vi "rethinkdb_json_tokenize_next.vi"(9 "offset (0)":i32, 11 "json":string) -> (1 "offset past token":i32, 2 "arg":string, 3 "token":T1)   [LabVIEW 2017]
uses:
  rethinkdb_json_token.ctl
  <vilib>/regexp/Match Regular Expression.xnode
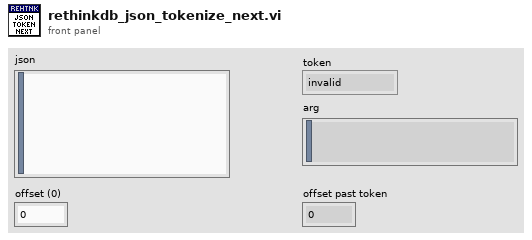
[diagram p1: front panel]
types:
  T1 = typedef "rethinkdb_json_token.ctl" = enum8{"invalid", "null", "boolean", "decimal", "float", "string", "key", "comma", "object_start", "object_end", "array_start", "array_end", "end"}
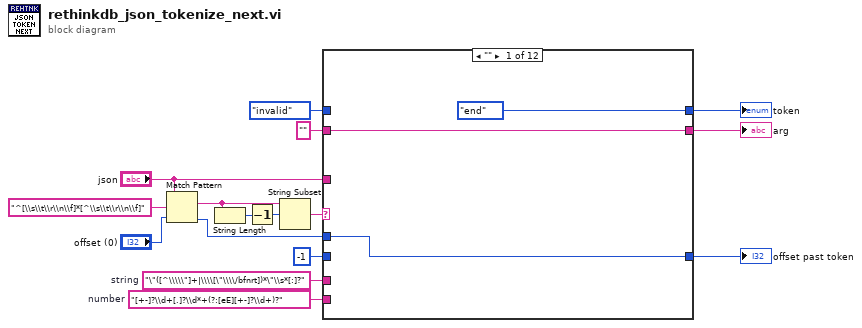
[diagram p0: block diagram]
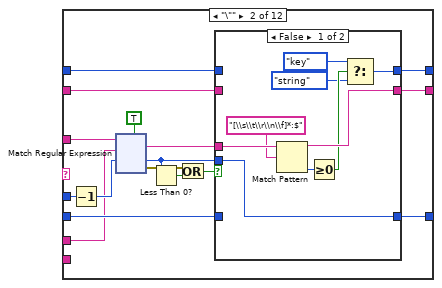
[diagram p2: hidden frame]
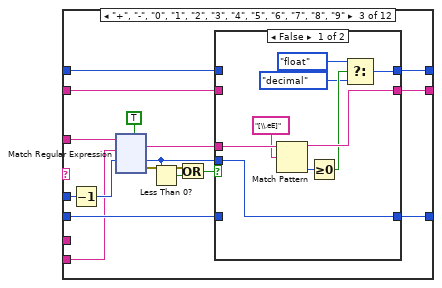
[diagram p4: hidden frame]
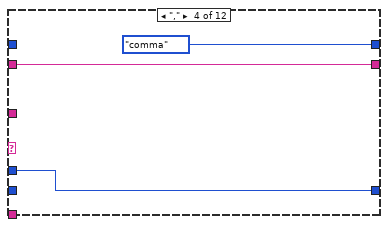
[diagram p6: hidden frame]
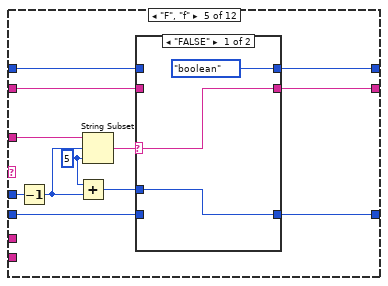
[diagram p7: hidden frame]
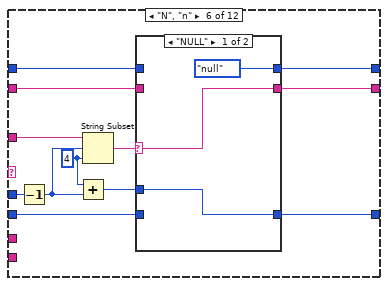
[diagram p9: hidden frame]
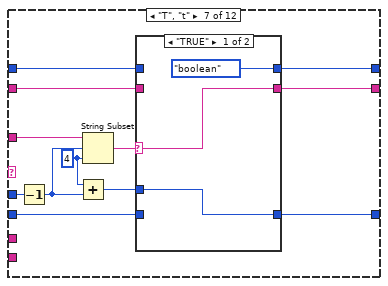
[diagram p11: hidden frame]
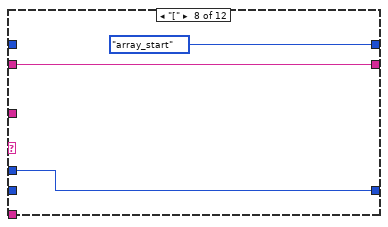
[diagram p13: hidden frame]
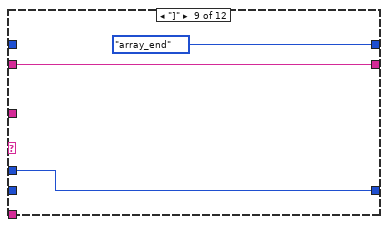
[diagram p14: hidden frame]
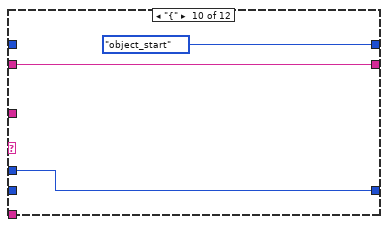
[diagram p15: hidden frame]
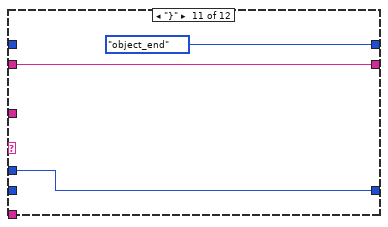
[diagram p16: hidden frame]
diagram:
  w1 = "[+-]?\\d+[.]?\\d*+(?:[eE][+-]?\\d+)?"  # number
  w2 = "\"([^\\\\\"]+|\\\\[\"\\\\/bfnrt])*\"\\s*[:]?"  # string
  n1 = Match Pattern(string="json", regular expression="^[\\s\\t\\r\\n\\f]*[^\\s\\t\\r\\n\\f]", offset (0)="offset (0)") -> (match substring=w13:string, offset past match=w8:i32)  [unwired: 2 out]
  n2 = String Length(string=w13) -> (length=w14:i32)
  n3 = Decrement(x=w14) -> (x-1=w12:i32)
  n4 = String Subset(string=w13, offset (0)=w12) -> (substring=w11:string)  [unwired: 1 in]
  n5 = case shown="\"\"" w11 {
    tunnel: [rethinkdb_json_token."end" ("token") w24 w166 rethinkdb_json_token."comma" ("token") w308 w326 w344 rethinkdb_json_token."array_start" ("token") rethinkdb_json_token."array_end" ("token") rethinkdb_json_token."object_start" ("token") rethinkdb_json_token."object_end" ("token") w375] -> w10
    tunnel: rethinkdb_json_token."invalid" ("token") -> [_ w23 w165 _ w307 w325 w343 _ _ _ _ w375]
    tunnel: w8 -> [w17 w33 w175 w304 w317 w335 w353 w361 w364 w367 w370 _]
    tunnel: [w17 w28 w170 w304 w312 w330 w348 w361 w364 w367 w370 w374] -> w7
    tunnel: -1 ("offset past match") -> [_ w27 w169 _ w311 w329 w347 _ _ _ _ w374]
    tunnel: [w19 w26 w168 w306 w310 w328 w346 w363 w366 w369 w372 w373] -> w5
    tunnel: "" -> [w19 w25 w167 w306 w309 w327 w345 w363 w366 w369 w372 w373]
    tunnel: "json" -> [_ w35 w177 _ w318 w336 w354 _ _ _ _ _]
    tunnel: w2 -> [_ w20 _ _ _ _ _ _ _ _ _ _]
    tunnel: w1 -> [_ _ w162 _ _ _ _ _ _ _ _ _]
    frame "" {
    }
    frame "\"" {
      n6 = Decrement(x=w33) -> (x-1=w32:i32)
      n7 = xnode "Match Regular Expression"("input string"=w35, "regular expression"=w20, "offset (0)"=w32, "multiline? (F)"=TRUE) -> ("whole match"=w21:string, "offset past match"=w22:i32, "error out"=w31:errorcluster)  [unwired: 2 in, 2 out]
      n8 = Less Than 0?(x=w22) -> (x < 0?=w30:bool)
      n9 = Or(x=w31, y=w30) -> (x .or. y?=w29:bool)
      n10 = case shown="False" w29 {
        tunnel: [w36 w47] -> w28
        tunnel: w27 -> [_ w47]
        tunnel: [w42 w46] -> w26
        tunnel: w25 -> [_ w46]
        tunnel: [w37 w45] -> w24
        tunnel: w23 -> [_ w45]
        tunnel: w22 -> [w36 _]
        tunnel: w21 -> [w44 _]
        frame False {
          n11 = Match Pattern(string=w44, regular expression="[\\s\\t\\r\\n\\f]*:$") -> (before substring=w42:string, offset past match=w41:i32)  [unwired: 1 in, 2 out]
          n12 = Greater Or Equal To 0?(x=w41) -> (x >= 0?=w40:bool)
          n13 = Select(t=rethinkdb_json_token."key" ("token"), s=w40, f=rethinkdb_json_token."string" ("token")) -> (s? t:f=w37:T1)
        }
        frame True {
        }
      }
    }
    frame "+", "-", "0", "1", "2", "3", "4", "5", "6", "7", "8", "9" {
      n14 = Decrement(x=w175) -> (x-1=w174:i32)
      n15 = xnode "Match Regular Expression"("input string"=w177, "regular expression"=w162, "offset (0)"=w174, "multiline? (F)"=TRUE) -> ("whole match"=w163:string, "offset past match"=w164:i32, "error out"=w173:errorcluster)  [unwired: 2 in, 2 out]
      n16 = Less Than 0?(x=w164) -> (x < 0?=w172:bool)
      n17 = Or(x=w173, y=w172) -> (x .or. y?=w171:bool)
      n18 = case shown="False" w171 {
        tunnel: [w178 w189] -> w170
        tunnel: w169 -> [_ w189]
        tunnel: [w184 w188] -> w168
        tunnel: w167 -> [_ w188]
        tunnel: [w179 w187] -> w166
        tunnel: w165 -> [_ w187]
        tunnel: w164 -> [w178 _]
        tunnel: w163 -> [w186 _]
        frame False {
          n19 = Match Pattern(string=w186, regular expression="[\\.eE]") -> (before substring=w184:string, offset past match=w183:i32)  [unwired: 1 in, 2 out]
          n20 = Greater Or Equal To 0?(x=w183) -> (x >= 0?=w182:bool)
          n21 = Select(t=rethinkdb_json_token."float" ("token"), s=w182, f=rethinkdb_json_token."decimal" ("token")) -> (s? t:f=w179:T1)
        }
        frame True {
        }
      }
    }
    frame "," {
    }
    frame "F", "f" {
      w315 = 5 ("length (rest)")
      n22 = Decrement(x=w317) -> (x-1=w316:i32)
      n23 = Add(x=w315, y=w316) -> (x+y=w314:i32)
      n24 = String Subset(string=w318, offset (0)=w316, length (rest)=w315) -> (substring=w313:string)
      n25 = case shown="\"FALSE\"" w313 {
        selector: w313 -> [w320 _]
        tunnel: w314 -> [w319 _]
        tunnel: [w319 w324] -> w312
        tunnel: w311 -> [_ w324]
        tunnel: [w320 w323] -> w310
        tunnel: w309 -> [_ w323]
        tunnel: [rethinkdb_json_token."boolean" ("token") w322] -> w308
        tunnel: w307 -> [_ w322]
        frame "FALSE" {
        }
        frame Default {
        }
      }
    }
    frame "N", "n" {
      w333 = 4 ("length (rest)")
      n26 = Decrement(x=w335) -> (x-1=w334:i32)
      n27 = Add(x=w333, y=w334) -> (x+y=w332:i32)
      n28 = String Subset(string=w336, offset (0)=w334, length (rest)=w333) -> (substring=w331:string)
      n29 = case shown="\"NULL\"" w331 {
        selector: w331 -> [w338 _]
        tunnel: w332 -> [w337 _]
        tunnel: [w337 w342] -> w330
        tunnel: w329 -> [_ w342]
        tunnel: [w338 w341] -> w328
        tunnel: w327 -> [_ w341]
        tunnel: [rethinkdb_json_token."null" ("token") w340] -> w326
        tunnel: w325 -> [_ w340]
        frame "NULL" {
        }
        frame Default {
        }
      }
    }
    frame "T", "t" {
      w351 = 4 ("length (rest)")
      n30 = Decrement(x=w353) -> (x-1=w352:i32)
      n31 = Add(x=w351, y=w352) -> (x+y=w350:i32)
      n32 = String Subset(string=w354, offset (0)=w352, length (rest)=w351) -> (substring=w349:string)
      n33 = case shown="\"TRUE\"" w349 {
        selector: w349 -> [w356 _]
        tunnel: w350 -> [w355 _]
        tunnel: [w355 w360] -> w348
        tunnel: w347 -> [_ w360]
        tunnel: [w356 w359] -> w346
        tunnel: w345 -> [_ w359]
        tunnel: [rethinkdb_json_token."boolean" ("token") w358] -> w344
        tunnel: w343 -> [_ w358]
        frame "TRUE" {
        }
        frame Default {
        }
      }
    }
    frame "[" {
    }
    frame "]" {
    }
    frame "{" {
    }
    frame "}" {
    }
    frame Default {
    }
  }
  "token" <- w10
  "arg" <- w5
  "offset past token" <- w7
